vi "DriverStationGetCommands.vi"() -> ()   [LabVIEW 2020]
doc: "This VI receives instructions from the driver and manipulator controls, but only in certain robot modes. Specifically, these instructions are received while the robot is either \"running autonomously\" or in Super Test Mode. In all other robot modes, no instructions are received via the driver station. Instead they are output by the Autonomous Sequencer or completely disabled."
uses:
  refnums.vi
  GRNF_Joystick.vi
  dscommands.vi
panel:
  in  "Buttons":bool[](array[boolean])=[FALSE, FALSE, FALSE, FALSE, FALSE, FALSE, FALSE, FALSE, FALSE, FALSE]
  in  "Right Trigger":dbl(slide) min=0.0 max=1.0 scale=0.0..1.0
  in  "Left Trigger":dbl(slide) min=0.0 max=1.0 step=0.1 scale=0.0..1.0
  in  "Right Joystick X":dbl(slide) scale=-1.0..1.0
  in  "Enable Joystick Control Override":bool
  in  "Joystick Left X":dbl(slide) scale=-1.0..1.0
  in  "Joystick Left Y":dbl(slide) scale=1.0..-1.0
  in  "Joystick Right Y":dbl(slide) scale=1.0..-1.0
  # "Left Thumbstick"
  # "Right Thumbstick"
  # "Driver A"
  # "Driver B"
  # "Driver X"
  # "Driver Y"
  # "Driver Left Bumper"
  # "Driver Right Bumper"
  # "Driver View"
  # "Driver Menu"
  # "Driver Left Joystick Button"
  # "Driver Right Joystick Button"
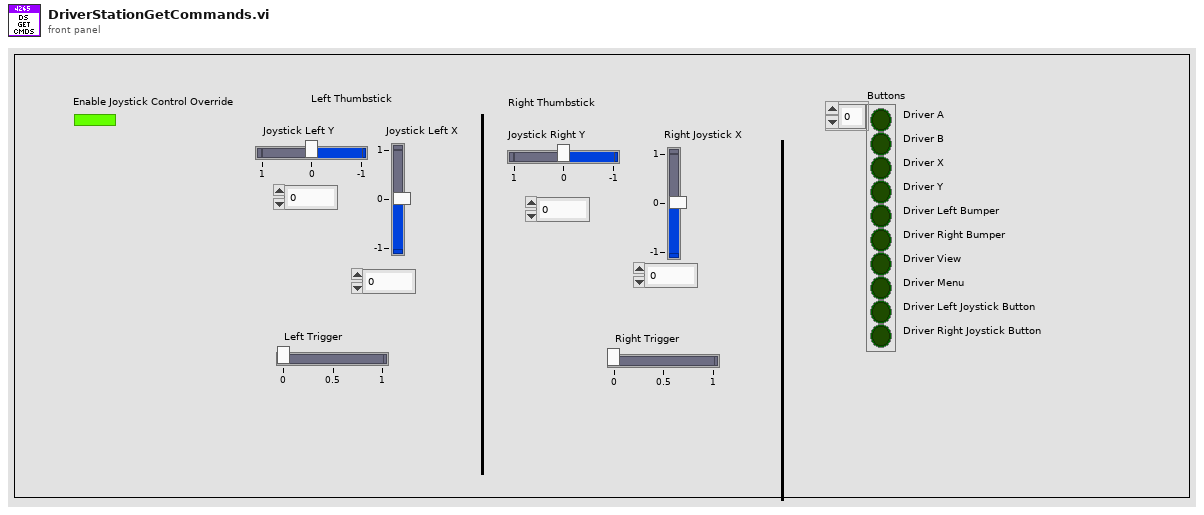
[diagram p1: front panel]
types:
  T1 = typedef "WPI_JoystickDevRef.ctl" = cluster{"Device":T2}
  T2 = typedef "WPI_JoystickDeviceEnum.ctl" = enum16{"USB 0", "USB 1", "USB 2", "USB 3", "USB 4", "USB 5"}
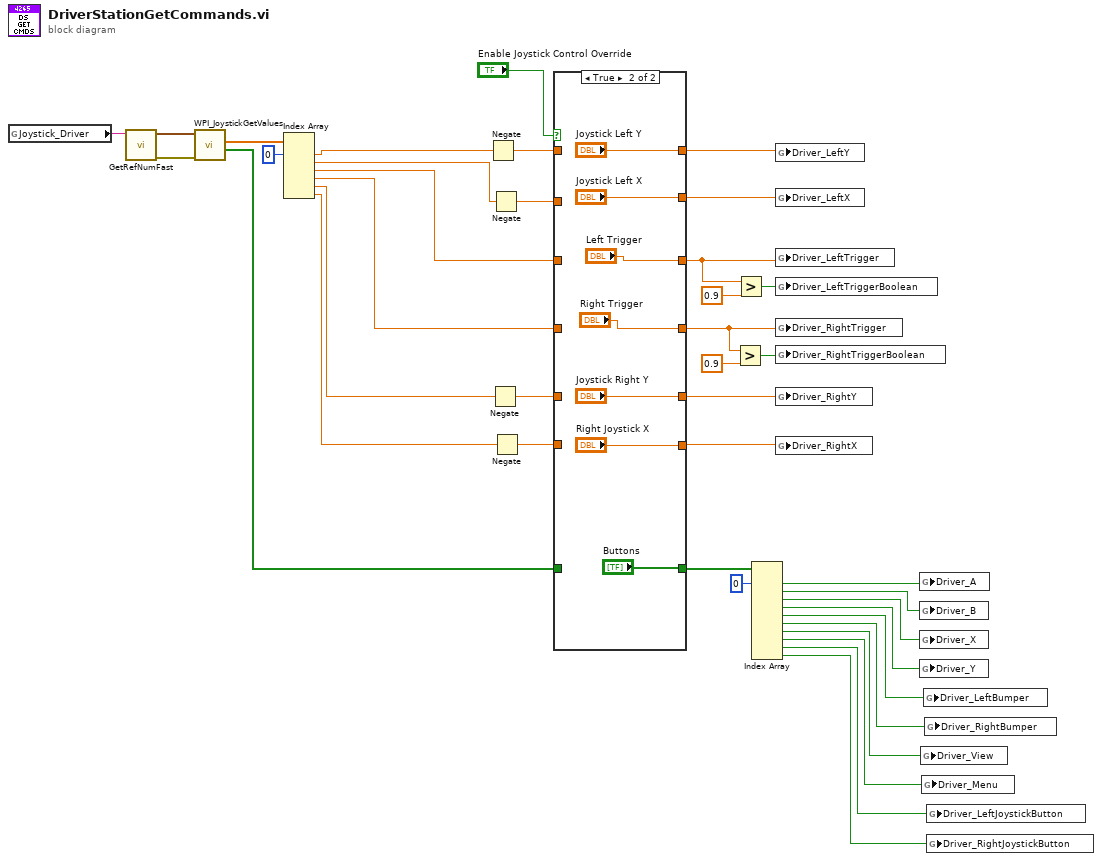
[diagram p0: block diagram]
diagram:
  n1 = global read "refnums.vi" "Joystick_Driver"() -> (w24:string)
  n2 = call-poly "GetRefNumFast.vi"("RefNum Name"=w24) -> ("Error"=w25:errorcluster, "Device Reference"=w26:T1)  [unwired: 5 in]
  n3 = call <vilib>:"WPI_JoystickGetValues.vi"("error in (no error)"=w25, "JoystickDevRef"=w26) -> ("Buttons"=w2:bool[], "Axes"=w39:dbl[])  [unwired: 5 in, 3 out]
  n4 = Index Array(array=w39, index #1=0 ("index")) -> (element #1=w23:dbl, element #2=w22:dbl, element #3=w18:dbl, element #4=w19:dbl, element #5=w20:dbl, element #6=w21:dbl)  [unwired: 5 in]
  n5 = Negate(x=w23) -> (-x=w15:dbl)
  n6 = Negate(x=w20) -> (-x=w5:dbl)
  n7 = Negate(x=w22) -> (-x=w14:dbl)
  n8 = Negate(x=w21) -> (-x=w4:dbl)
  n9 = case shown="True" "Enable Joystick Control Override" {
    tunnel: w18 -> [w44 _]
    tunnel: [w46 "Joystick Left Y"] -> w16
    tunnel: w15 -> [w46 _]
    tunnel: [w45 "Joystick Left X"] -> w13
    tunnel: w14 -> [w45 _]
    tunnel: [w44 "Left Trigger"] -> w8
    tunnel: w19 -> [w43 _]
    tunnel: [w43 "Right Trigger"] -> w7
    tunnel: [w42 "Joystick Right Y"] -> w6
    tunnel: w5 -> [w42 _]
    tunnel: [w41 "Right Joystick X"] -> w3
    tunnel: w4 -> [w41 _]
    tunnel: w2 -> [w40 _]
    tunnel: [w40 "Buttons"] -> w1
    frame False {
    }
    frame True {
    }
  }
  n10 = Greater?(x=w7, y=0.9) -> (0:w10:bool)
  n11 = Greater?(x=w8, y=0.9) -> (0:w9:bool)
  n12 = Index Array(array=w1, index #1=0 ("index")) -> (element #1=w36:bool, element #2=w35:bool, element #3=w34:bool, element #4=w33:bool, element #5=w32:bool, element #6=w31:bool, element #7=w30:bool, element #8=w29:bool, element #9=w28:bool, element #10=w27:bool)  [unwired: 9 in]
  n13 = global write "dscommands.vi" "Driver_LeftY"(w16) -> ()
  n14 = global write "dscommands.vi" "Driver_LeftX"(w13) -> ()
  n15 = global write "dscommands.vi" "Driver_LeftTrigger"(w8) -> ()
  n16 = global write "dscommands.vi" "Driver_LeftTriggerBoolean"(w9) -> ()
  n17 = global write "dscommands.vi" "Driver_RightTrigger"(w7) -> ()
  n18 = global write "dscommands.vi" "Driver_RightTriggerBoolean"(w10) -> ()
  n19 = global write "dscommands.vi" "Driver_RightY"(w6) -> ()
  n20 = global write "dscommands.vi" "Driver_RightX"(w3) -> ()
  n21 = global write "dscommands.vi" "Driver_A"(w36) -> ()
  n22 = global write "dscommands.vi" "Driver_B"(w35) -> ()
  n23 = global write "dscommands.vi" "Driver_X"(w34) -> ()
  n24 = global write "dscommands.vi" "Driver_Y"(w33) -> ()
  n25 = global write "dscommands.vi" "Driver_View"(w30) -> ()
  n26 = global write "dscommands.vi" "Driver_Menu"(w29) -> ()
  n27 = global write "dscommands.vi" "Driver_LeftBumper"(w32) -> ()
  n28 = global write "dscommands.vi" "Driver_RightBumper"(w31) -> ()
  n29 = global write "dscommands.vi" "Driver_LeftJoystickButton"(w28) -> ()
  n30 = global write "dscommands.vi" "Driver_RightJoystickButton"(w27) -> ()
